vi "SaveItfMessage.vi"(8 "error in (no error)":errorcluster caption="entrée d'erreur (pas d'erreur)", 11 "cheminIn":path) -> (0 "error out":errorcluster caption="sortie d'erreur", 1 "Cancel Out":bool, 2 "StartITF Out":bool=TRUE, 3 "CheminOut":path)   [LabVIEW 2010, in "Interface.lvclass"]
uses:
  Interface.lvclass
panel:
  in  "Cancel":bool
  in  "Save":bool
  in  "StartITF":bool=TRUE
  # "Sauvegarder le projet courrant sous:"
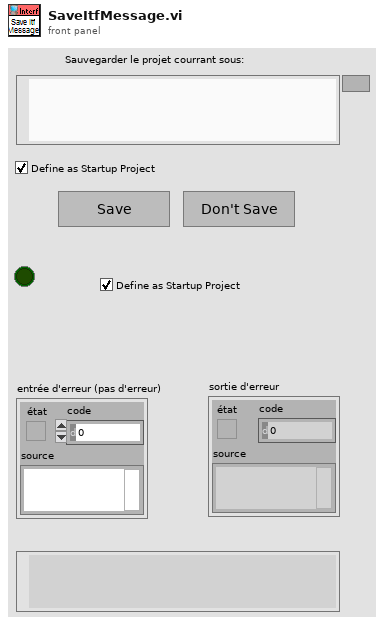
[diagram p1: front panel]
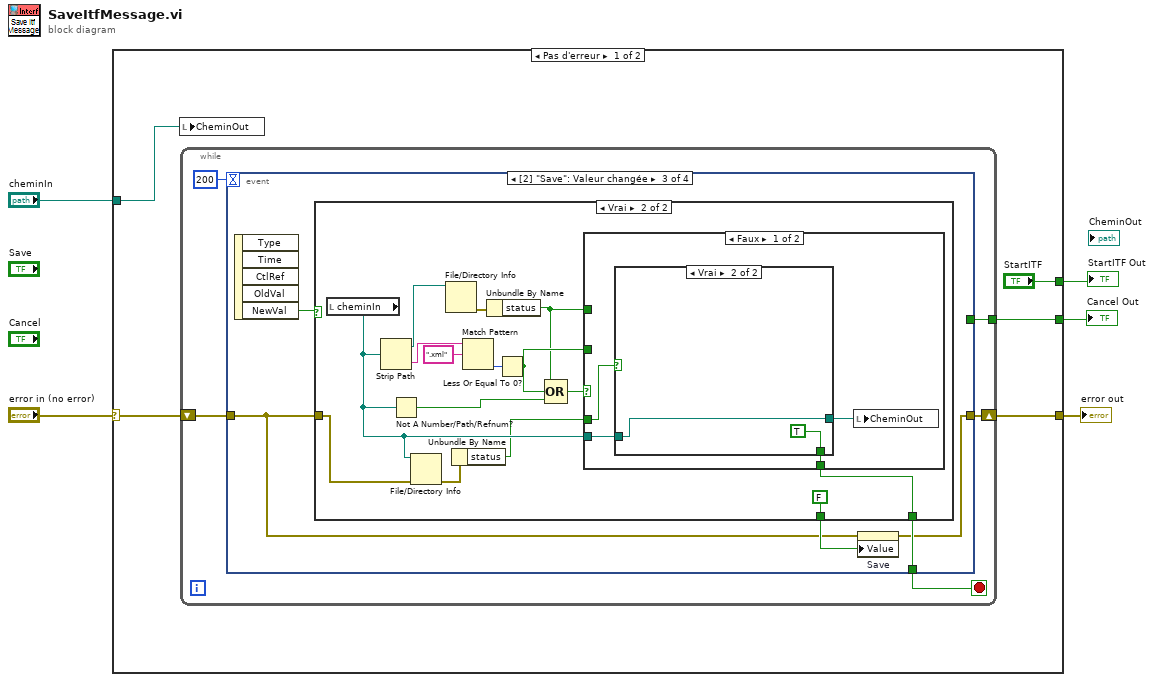
[diagram p0: block diagram]
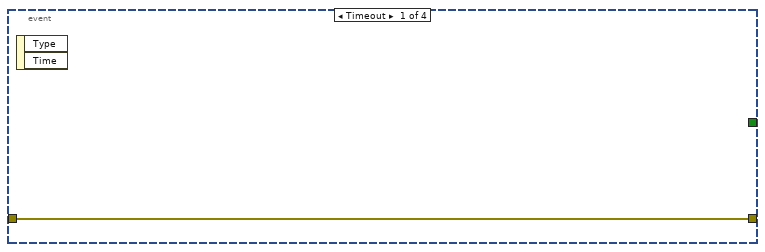
[diagram p2: hidden frame]
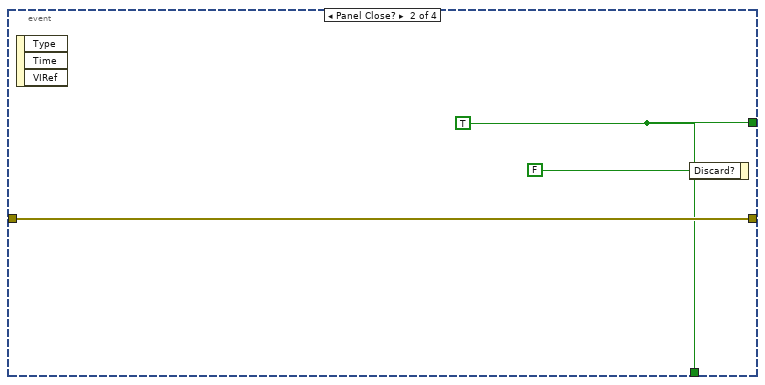
[diagram p3: hidden frame]
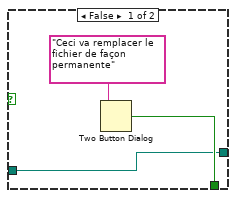
[diagram p5: hidden frame]
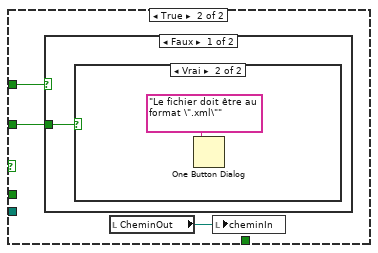
[diagram p6: hidden frame]
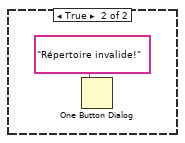
[diagram p8: hidden frame]
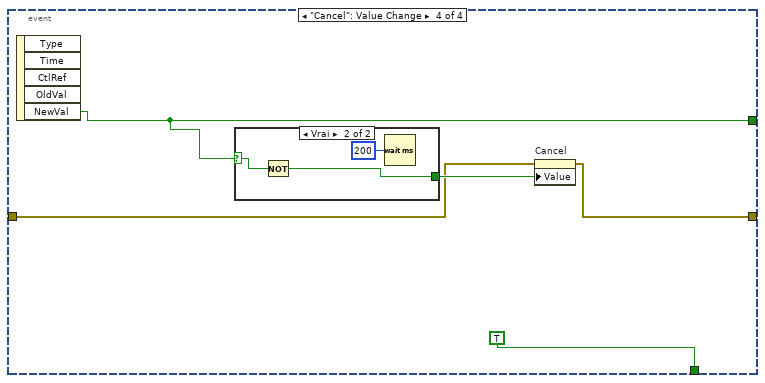
[diagram p9: hidden frame]
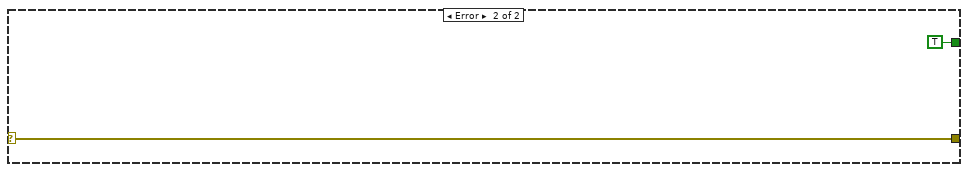
[diagram p11: hidden frame]
diagram:
  n1 = case shown="Pas d'erreur" "error in (no error)" {
    selector: "error in (no error)" -> [w7 w65]
    tunnel: [w10 w65] -> w4
    tunnel: [w9 TRUE] -> w2
    tunnel: "cheminIn" -> [w8 _]
    tunnel: ["StartITF" _] -> w1
    frame No Error {
      n2 = local write "CheminOut"(w8) -> ()
      n3 = while {
        shift-right: [w13] -> w10
        shift-left: w7 -> [w14]
        tunnel: [w12] -> w9
        stop <- w11 stop-if-true
        n4 = event shown="[2] \"Save\": Valeur changée" {
          selector: _ -> [_ _ _ _]
          dyn-events: _ -> [_ _ _ _]
          timeout: 200 -> [_ _ _ _]
          tunnel: w14 -> [w16 w18 w20 w56]
          tunnel: [w16 w18 w21 w55] -> w13
          tunnel: [_ w17 _ w58] -> w12
          tunnel: [_ w17 w23 TRUE] -> w11
          event Timeout {
            n5 = event-data() -> ()  [unwired: 1 in, 2 out]
          }
          event Panel Close? {
            w17 = TRUE
            n6 = event-data() -> ()  [unwired: 1 in, 3 out]
            n7 = event-data("Discard?"=FALSE ("Rejeter ?")) -> ()  [unwired: 1 in, 1 out]
          }
          event "Save": Value Change {
            n8 = event-data() -> ("NewVal"=w24:bool)  [unwired: 1 in, 4 out]
            n9 = case shown="Vrai" w24 {
              tunnel: [_ FALSE] -> w22
              tunnel: w20 -> [_ w25]
              tunnel: [_ w26] -> w23
              frame False {
              }
              frame True {
                n10 = local read "cheminIn"() -> (w33:path)
                n11 = Strip Path(path=w33) -> (stripped path=w30:path, name=w39:string)
                n12 = Not A Number/Path/Refnum?(number/path/refnum=w33) -> (NaN/Path/Refnum?=w36:bool)
                n13 = File/Directory Info(path=w33, error in=w25) -> (error out=w32:errorcluster)  [unwired: 6 out]
                n14 = File/Directory Info(path=w30) -> (error out=w29:errorcluster)  [unwired: 1 in, 6 out]
                n15 = Unbundle By Name(w32) -> ("status"=w31:bool)
                n16 = Match Pattern(string=w39, regular expression=".xml" ("expression régulière")) -> (offset past match=w37:i32)  [unwired: 1 in, 3 out]
                n17 = Unbundle By Name(w29) -> ("status"=w28:bool)
                n18 = Less Or Equal To 0?(x=w37) -> (x <= 0?=w34:bool)
                n19 = Compound Arithmetic op=OR(w28, w34, w36) -> (w35:bool)
                n20 = case shown="Faux" w35 {
                  tunnel: w33 -> [w43 _]
                  tunnel: w34 -> [_ w51]
                  tunnel: w31 -> [w40 _]
                  tunnel: w28 -> [_ w49]
                  tunnel: [w42 _] -> w26
                  frame False {
                    n21 = case shown="Vrai" w40 {
                      tunnel: w43 -> [w44 w47]
                      tunnel: [w45 TRUE] -> w42
                      tunnel: [w44 w47] -> w41
                      frame False {
                        n22 = Two Button Dialog(message="Ceci va remplacer le fichier de façon permanente" ("pattern label")) -> (T button?=w45:bool)  [unwired: 2 in]
                      }
                      frame True {
                      }
                    }
                    n23 = local write "CheminOut"(w41) -> ()
                  }
                  frame True {
                    n24 = case shown="Faux" w49 {
                      tunnel: w51 -> [w52 _]
                      frame False {
                        n25 = case shown="Vrai" w52 {
                          frame False {
                          }
                          frame True {
                            n26 = One Button Dialog(message="Le fichier doit être au format \".xml\"" ("pattern label")) -> ()  [unwired: 1 in, 1 out]
                          }
                        }
                      }
                      frame True {
                        n27 = One Button Dialog(message="Répertoire invalide!" ("pattern label")) -> ()  [unwired: 1 in, 1 out]
                      }
                    }
                    n28 = local read "CheminOut"() -> (w50:path)
                    n29 = local write "cheminIn"(w50) -> ()
                  }
                }
              }
            }
            n30 = property on="Save" class="Bool (strict)"(error in=w20, "Value"=w22) -> (error out=w21:errorcluster)  [unwired: 1 in, 1 out]
          }
          event "Cancel": Value Change {
            n31 = event-data() -> ("NewVal"=w58:bool)  [unwired: 1 in, 4 out]
            n32 = case shown="Vrai" w58 {
              selector: w58 -> [w60 w63]
              tunnel: [w60 w61] -> w57
              frame False {
              }
              frame True {
                n33 = Not(x=w63) -> (.not. x?=w61:bool)
                n34 = Wait (ms)(milliseconds to wait=u32 200 ("attente (ms)")) -> ()  [unwired: 1 out]
              }
            }
            n35 = property on="Cancel" class="Bool (strict)"(error in=w56, "Value"=w57) -> (error out=w55:errorcluster)  [unwired: 1 in, 1 out]
          }
        }
      }
    }
    frame Error {
    }
  }
  "error out" <- w4
  "Cancel Out" <- w2
  "StartITF Out" <- w1
